vi "Formula Replace Pi.vi"(5 "Formula In":string="sin(5 * Pi* t)") -> (2 "Formula Out":string)   [LabVIEW 2019, in "ObjectSettings.lvclass"]
uses:
  ObjectSettings.lvclass
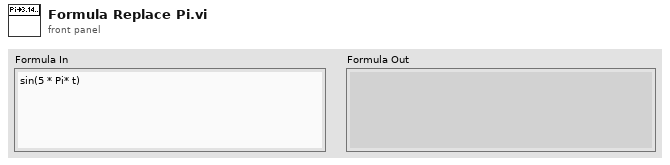
[diagram p1: front panel]
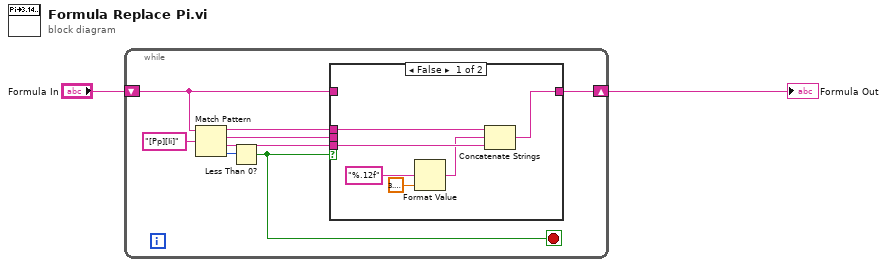
[diagram p0: block diagram]
diagram:
  n1 = while {
    shift-right: [w4] -> w1
    shift-left: "Formula In" -> [w5]
    stop <- w3 stop-if-true
    n2 = Match Pattern(string=w5, regular expression="[Pp][Ii]") -> (before substring=w8:string, match substring=w7:string, after substring=w6:string, offset past match=w9:i32)  [unwired: 1 in]
    n3 = Less Than 0?(x=w9) -> (x < 0?=w3:bool)
    n4 = case shown="False" w3 {
      tunnel: w8 -> [w16 _]
      tunnel: w7 -> [_ _]
      tunnel: w6 -> [w15 _]
      tunnel: w5 -> [_ w17]
      tunnel: [w14 w17] -> w4
      frame False {
        n5 = Format Value(format string="%.12f", value (0)=3.141592653589793) -> (output string=w12:string)  [unwired: 1 in]
        n6 = Concatenate Strings(w16, w12, w15) -> (w14:string)
      }
      frame True {
      }
    }
  }
  "Formula Out" <- w1
